vi "LaunchAutoMode.vi"(7 "TestSettings":T1, 8 "error in (no error)":errorcluster, 9 "Subpanel":refnum<vi>, 10 "MainQueue":refnum<queue>, 11 "AutoModeQueue":refnum<queue>) -> (0 "error out":errorcluster)   [LabVIEW 2019, in "MainController.lvlib"]
uses:
  MainController.lvlib
  AutoMode/Cluster - AutoModeMessage.ctl
  AutoMode/Enum - AutoModeState.ctl
  Cluster - MainControllerMessage.ctl
  Enum - MainState.ctl
  Cluster - TestSettings.ctl
  AutoMode/Cluster - AutoModeData.ctl
  Cluster - HardwareConfiguration.ctl
  Cluster - TestResults.ctl
  AutoMode/AutoMode.vi
  support/User Interface/UserInterface.lvlib
  AutoMode/AutoMode.lvlib
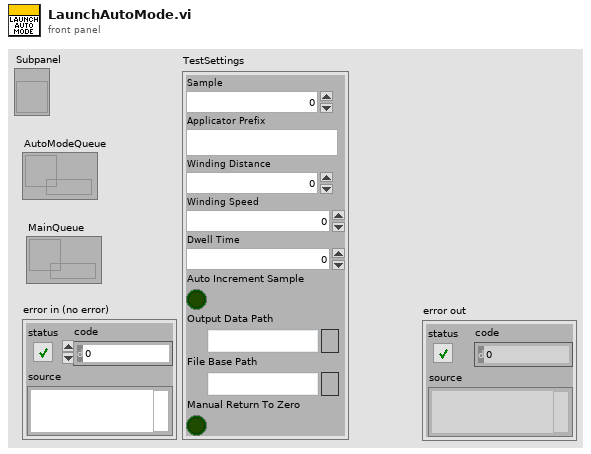
[diagram p1: front panel]
types:
  T1 = typedef "MainController.lvlib/Cluster - TestSettings.ctl" = cluster{"Sample":u32, "Applicator Prefix":string, "Winding Distance":dbl, "Winding Speed":dbl, "Dwell Time":dbl, "Auto Increment Sample":bool, "Output Data Path":path, "File Base Path":path, "Manual Return To Zero":bool}
  T2 = typedef "AutoMode.lvlib/Cluster - AutoModeData.ctl" = cluster{"DataDisplayQueue":refnum<queue>, "StepStartTime":timestamp, "TestSettings":T1, "Hardware Configuration":T3, "TestResults":T4, "ElapsedTime":dbl, "IsFirstSample":bool, "UIRefs":map{string, refnum<vi>}, "SelfQueue":refnum<queue>, "MainQueue":refnum<queue>}
  T3 = typedef "MainController.lvlib/Cluster - HardwareConfiguration.ctl" = cluster{"Mark10COM":refnum<visa-resource-name>, "IsConnected":bool}
  T4 = typedef "MainController.lvlib/Cluster - TestResults.ctl" = cluster{"AcquiredData":dbl[][], "TestStartTime":timestamp}
  T5 = typedef "AutoMode.lvlib/Enum - AutoModeState.ctl" = enum16{"Initialize", "Idle", "UpdateConfig", "BroadcastSettings", "Start", "CheckValidReportPath", "Winding", "WaitForWinding", "Unwind", "WaitForUnwind", "Stop", "Abort", "WriteDataToFile", "EventTriggered", "GenerateFilePath", "ZeroPosition", "GotoZero", "Error", "Exit"}
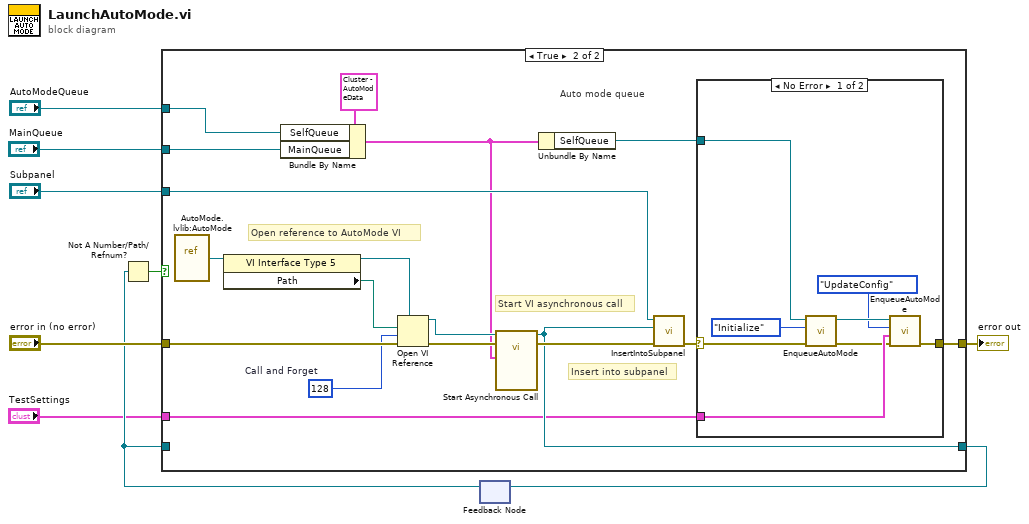
[diagram p0: block diagram]
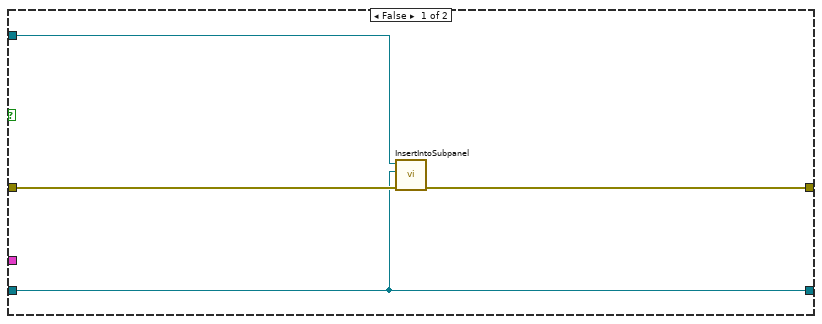
[diagram p2: hidden frame]
diagram:
  n1 = feedback #1() -> (w5:refnum<vi>)  [unwired: 1 in]
  n2 = Not A Number/Path/Refnum?(number/path/refnum=w5) -> (NaN/Path/Refnum?=w4:bool)
  n3 = case shown="True" w4 {
    tunnel: "error in (no error)" -> [w13 w31]
    tunnel: "Subpanel" -> [w12 w29]
    tunnel: [w10 w25] -> w7
    tunnel: [w11 w21] -> w6
    tunnel: w5 -> [w11 _]
    tunnel: "AutoModeQueue" -> [_ w16]
    tunnel: "MainQueue" -> [_ w17]
    tunnel: "TestSettings" -> [_ w19]
    frame False {
      n4 = call "InsertIntoSubpanel.vi"("error in (no error)"=w13, "VI Ref"=w11, "Subpanel"=w12) -> ("error out"=w10:errorcluster)  [unwired: 8 in]
    }
    frame True {
      w23 = 128  # Call and Forget
      # "Auto mode queue"
      # "Insert into subpanel"
      # "Start VI asynchronous call"
      # "Open reference to AutoMode VI"
      n5 = vi-ref "AutoMode.lvlib:AutoMode.vi"() -> (w24:refnum<vi>)
      n6 = property class="VI Interface Type 5"(reference=w24) -> (reference out=w20:refnum<vi>, "Path"=w30:path)  [unwired: 1 in, 1 out]
      n7 = Bundle By Name(cluster=T2 {"DataDisplayQueue"=refnum, "StepStartTime"=timestamp(0 s since 1904-01-01), "TestSettings"={"Sample"=0, "Applicator Prefix"="", "Winding Distance"=0.0, "Winding Speed"=0.0, "Dwell Time"=0.0, "Auto Increment Sample"=FALSE, "Output Data Path"=path "", "File Base Path"=path "", "Manual Return To Zero"=FALSE}, "Hardware Configuration"={"Mark10COM"="", "IsConnected"=FALSE}, "TestResults"={"AcquiredData"=[], "TestStartTime"=timestamp(0 s since 1904-01-01)}, "ElapsedTime"=0.0, "IsFirstSample"=FALSE, "UIRefs"={}, "SelfQueue"=refnum, "MainQueue"=refnum} ("AutoData"), "SelfQueue"=w16, "MainQueue"=w17) -> (w15:T2)
      n8 = Open VI Reference(type specifier VI Refnum (for type only)=w20, vi path=w30, options=w23, error in (no error)=w31) -> (vi reference=w28:refnum<vi>, error out=w27:errorcluster)  [unwired: 2 in]
      n9 = call-by-ref "Start Asynchronous Call"(reference=w28, error in=w27, "AutoModeData"=w15) -> (reference out=w21:refnum<vi>, error out=w22:errorcluster)  [unwired: 10 in, 1 out]
      n10 = Unbundle By Name(w15) -> ("SelfQueue"=w14:refnum<queue>)
      n11 = call "InsertIntoSubpanel.vi"("error in (no error)"=w22, "VI Ref"=w21, "Subpanel"=w29) -> ("error out"=w26:errorcluster)  [unwired: 8 in]
      n12 = case shown="No Error" w26 {
        selector: w26 -> [w39 w40]
        tunnel: [w32 w40] -> w25
        tunnel: w14 -> [w37 _]
        tunnel: w19 -> [w34 _]
        frame No Error {
          n13 = call "EnqueueAutoMode.vi"("error in (no error)"=w39, "AutoState"=Enum_-_AutoModeState."Initialize" ("CycleTestState"), "Queue in"=w37) -> ("error out"=w33:errorcluster, "queue out"=w36:refnum<queue>)  [unwired: 7 in]
          n14 = call "EnqueueAutoMode.vi"("error in (no error)"=w33, "Data"=w34, "AutoState"=Enum_-_AutoModeState."UpdateConfig" ("CycleTestState"), "Queue in"=w36) -> ("error out"=w32:errorcluster)  [unwired: 6 in, 1 out]
        }
        frame Error {
        }
      }
    }
  }
  "error out" <- w7
  n15 = feedback-in #1(w6) -> ()
